vi "滤波.vi"() -> ()   [LabVIEW 2014]
uses:
  <vilib>/Analysis/2dsp.llb/Real FFT.vi
  <vilib>/measure/macond.llb/FIR Filter for 1 Chan.vi
  <vilib>/measure/madcrms.llb/Basic Averaged DC-RMS for 1 Chan.vi
  <vilib>/measure/NI_MAPro.lvlib
  <vilib>/measure/NI_MABase.lvlib
  <vilib>/Analysis/NI_AALPro.lvlib
  <vilib>/Analysis/NI_AALBase.lvlib
panel:
  out "波形图 4":dbl[](graph)
  out "波形图 3":dbl[](graph)
  in  "cycles 3":dbl=1.0 caption="周期" format="%0.2f"
  in  "amplitude 3":dbl=1.0 caption="幅值" format="%0.2f"
  in  "cycles 2":dbl=1.0 caption="周期" format="%0.2f"
  in  "amplitude 2":dbl=1.0 caption="幅值" format="%0.2f"
  in  "cycles":dbl=1.0 caption="周期" format="%0.2f"
  in  "amplitude":dbl=1.0 caption="幅值" format="%0.2f"
  in  "sampling info":cluster{"Fs":dbl, "#s":dbl}={"Fs"=1000.0, "#s"=1000.0} caption="采样信息" {"Fs" format="%.2p"}
  in  "FIR filter specifications":T1={"Topology"=enum."Off", "Type"=enum."Lowpass", "#Taps"=50, "Lower PB"=100.0, "Upper PB"=0.0, "Lower SB"=200.0, "Upper SB"=0.0} caption="FIR滤波器规范" {"Lower SB" format="%0.2p"; "Upper SB" format="%0.2p"; "Lower PB" format="%0.2p"; "Upper PB" format="%0.2p"}
  in  "数值":dbl
  out "波形图 2":waveform(dbl)(graph)
  out "波形图":waveform(dbl)(graph)
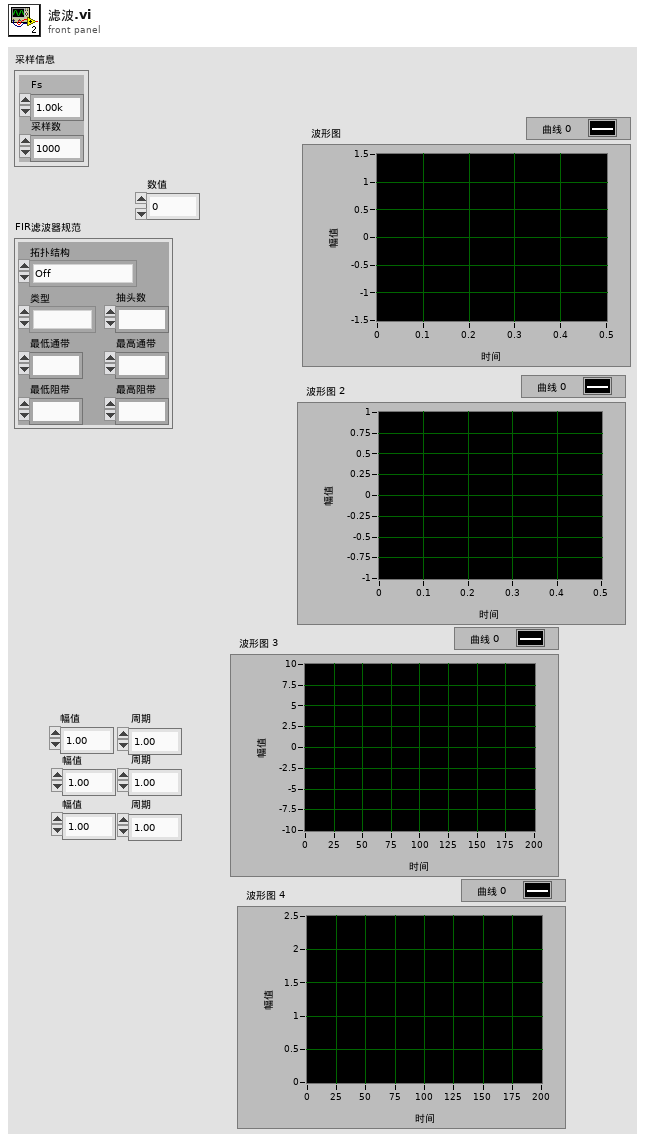
[diagram p1: front panel]
types:
  T1 = cluster{"Topology":enum16{"Off", "FIR by Specification", "Equi-ripple FIR", "Windowed FIR"}, "Type":enum16{"Lowpass", "Highpass", "Bandpass", "Bandstop"}, "#Taps":i32, "Lower PB":dbl, "Upper PB":dbl, "Lower SB":dbl, "Upper SB":dbl}
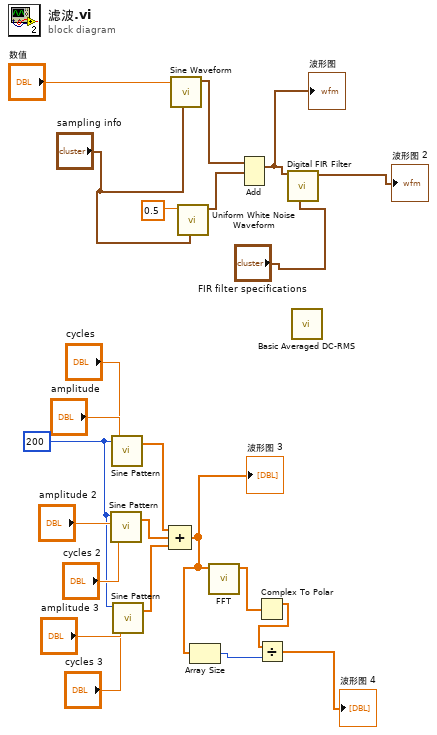
[diagram p0: block diagram]
diagram:
  w6 = 200
  n1 = call <vilib>:"Sine Pattern.vi"("cycles"="cycles 2", "amplitude"="amplitude 2", "samples"=w6) -> ("Sinusoidal Pattern"=w8:dbl[])  [unwired: 1 in, 1 out]
  n2 = call <vilib>:"Sine Pattern.vi"("cycles"="cycles", "amplitude"="amplitude", "samples"=w6) -> ("Sinusoidal Pattern"=w9:dbl[])  [unwired: 1 in, 1 out]
  n3 = call <vilib>:"Sine Pattern.vi"("cycles"="cycles 3", "amplitude"="amplitude 3", "samples"=w6) -> ("Sinusoidal Pattern"=w7:dbl[])  [unwired: 1 in, 1 out]
  n4 = Compound Arithmetic op=ADD(w9, w8, w7) -> (w1:dbl[])
  "波形图 3" <- w1
  n5 = call <vilib>:"Sine Waveform.vi"("sampling info"="sampling info", "frequency"="数值") -> ("signal out"=w19:waveform(dbl))  [unwired: 8 in, 1 out]
  n6 = call <vilib>:"Uniform White Noise Waveform.vi"("sampling info"="sampling info", "amplitude"=0.5) -> ("signal out"=w18:waveform(dbl))  [unwired: 8 in, 1 out]
  n7 = Array Size(array=w1) -> (size(s)=w2:i32)
  n8 = call-poly <vilib>:"FFT.vi"("X"=w1) -> ("FFT {X}"=w4:cdb[])  [unwired: 9 in, 1 out]
  n9 = Add(1:w18, 2:w19) -> (0:w20:waveform(dbl))  [unwired: 1 in, 1 out]
  "波形图" <- w20
  n10 = Complex To Polar(r * e^(i*theta)=w4) -> (r=w3:dbl[])  [unwired: 1 out]
  n11 = Divide(x=w3, y=w2) -> (x/y=→"波形图 4":dbl[])
  n12 = call-poly <vilib>:"Digital FIR Filter.vi"("FIR filter specifications"="FIR filter specifications", "signal in"=w20) -> ("signal out"=→"波形图 2":waveform(dbl))  [unwired: 7 in, 2 out]
  n13 = call-poly <vilib>:"Basic Averaged DC-RMS.vi"() -> ()  [unwired: 8 in, 4 out]
